vi "Get Category.vi"(8 "error in (no error)":errorcluster, 11 "EIP Tags editor node in":refnum<class "EIP Tags editor node.lvclass">) -> (0 "error out":errorcluster, 2 "Category":string, 3 "EIP Tags editor node out":refnum<class "EIP Tags editor node.lvclass">)   [LabVIEW 2013, in "EIP Tags editor node.lvclass"]
uses:
  EIP Tags editor node.lvclass
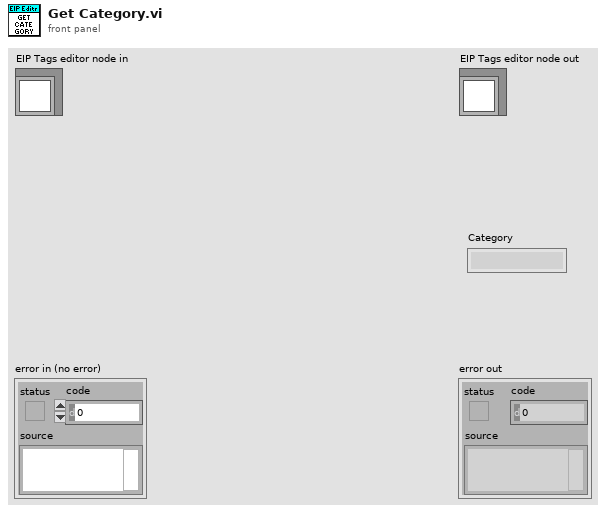
[diagram p1: front panel]
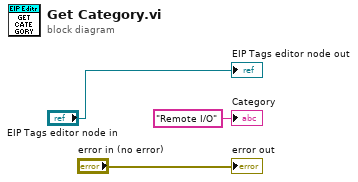
[diagram p0: block diagram]
diagram:
  "error out" <- "error in (no error)"
  "EIP Tags editor node out" <- "EIP Tags editor node in"
  "Category" <- "Remote I/O" ("Category")
